vi "Multiplexer_sendsubvi.vi"(3 "error in (no error)":errorcluster, 4 "Position":i32 min=0 max=7, 5 "Enum":T1(ring), 6 "VISA resource name":refnum<visa-resource-name>) -> (0 "error out":errorcluster, 1 "Response":string="answ 0\rjmp 1\rla 200\rla 35010001\rla -562\rla 358\rla 1246\rla 2136\rla 3038\rla 3926\rla 4816\rla 5718\rla -562\rla 358\rla 1246\rla 2136\rla 3038\rla 3926\rla 4816\rla 5718\ra 1\rv -70\rdelay 600\rgohix \rdelay 50\rla -562\rm \rdelay 50\rend:53\r\n", 2 "VISA resource name out":refnum<visa-resource-name>)   [LabVIEW 2018]
panel:
  out "concatenated string":string="GPROGSEQ\r"
  out "bytes read":u32=222
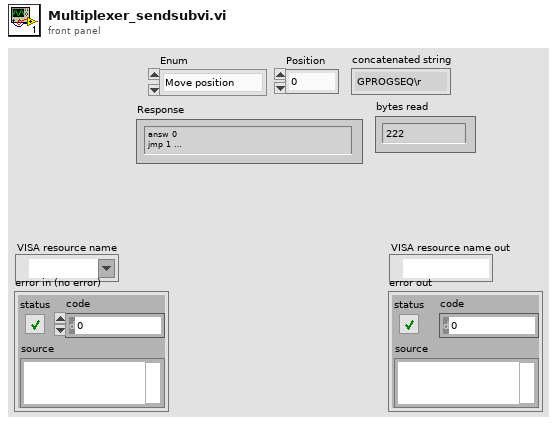
[diagram p1: front panel]
types:
  T1 = enum16{"Move position", "Get Status", "Get Program"}
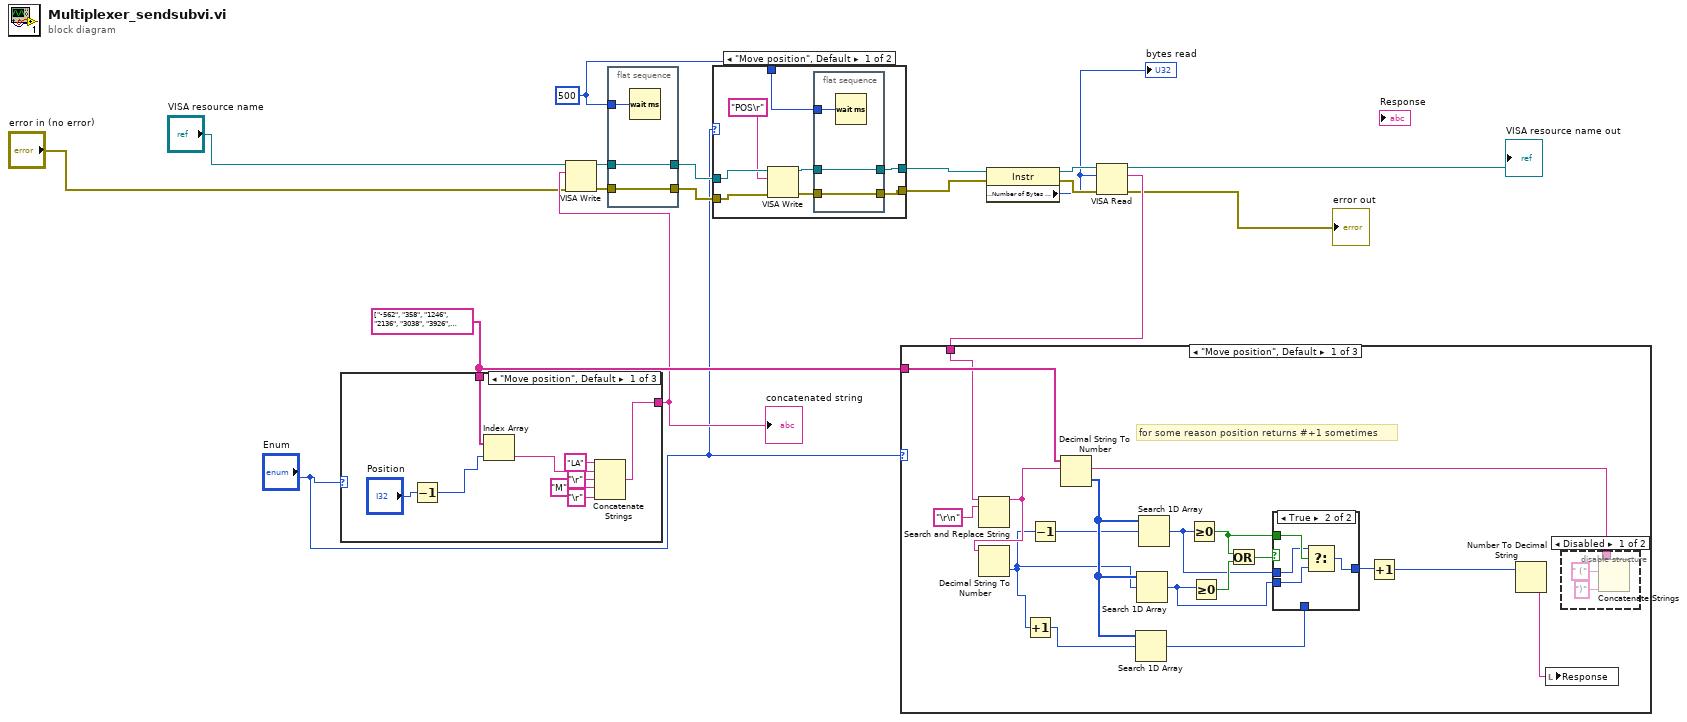
[diagram p0: block diagram]
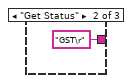
[diagram p7: hidden frame]
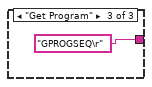
[diagram p8: hidden frame]
diagram:
  w12 = string[] ["-562", "358", "1246", "2136", "3038", "3926", "4816", "5718"]
  w7 = u32 500 ("delay before read (ms)")
  n1 = case shown="\"Move position\", Default" "Enum" {
    tunnel: [w22 "GST\r" "GPROGSEQ\r"] -> w11
    tunnel: w12 -> [w21 _ _]
    frame "Move position", Default {
      n2 = Decrement(x="Position") -> (x-1=w19:i32)
      n3 = Index Array(array=w21, index=w19) -> (element=w25:string)
      n4 = Concatenate Strings("LA" ("string"), w25, "\r" ("string"), "M" ("string"), "\r" ("string")) -> (w22:string)
    }
    frame "Get Status" {
    }
    frame "Get Program" {
    }
  }
  "concatenated string" <- w11
  n5 = VISA Write(VISA resource name="VISA resource name", write buffer=w11, error in (no error)="error in (no error)") -> (VISA resource name out=w17:refnum<visa-resource-name>, error out=w18:errorcluster)  [unwired: 1 out]
  n6 = flat-sequence {
    tunnel: w18 -> [w31]
    tunnel: [w31] -> w9
    tunnel: w17 -> [w30]
    tunnel: [w30] -> w10
    tunnel: w7 -> [w32]
    frame #0 {
      n7 = Wait (ms)(milliseconds to wait=w32) -> ()  [unwired: 1 out]
    }
  }
  n8 = case shown="\"Move position\", Default" "Enum" {
    tunnel: w10 -> [w40 w45]
    tunnel: w9 -> [w39 w44]
    tunnel: [w33 w44] -> w5
    tunnel: [w34 w45] -> w6
    tunnel: w7 -> [w37 _]
    frame "Move position", Default {
      n9 = VISA Write(VISA resource name=w40, write buffer="POS\r", error in (no error)=w39) -> (VISA resource name out=w36:refnum<visa-resource-name>, error out=w35:errorcluster)  [unwired: 1 out]
      n10 = flat-sequence {
        tunnel: w35 -> [w42]
        tunnel: [w42] -> w33
        tunnel: w36 -> [w41]
        tunnel: [w41] -> w34
        tunnel: w37 -> [w43]
        frame #0 {
          n11 = Wait (ms)(milliseconds to wait=w43) -> ()  [unwired: 1 out]
        }
      }
    }
    frame "Get Status" {
    }
  }
  n12 = property class="Instr"(reference=w6, error in=w5) -> (reference out=w16:refnum<visa-resource-name>, error out=w15:errorcluster, "Serial Settings:Number of Bytes at Serial Port"=w14:u32)
  "bytes read" <- w14
  n13 = VISA Read(VISA resource name=w16, byte count=w14, error in (no error)=w15) -> (VISA resource name out=→"VISA resource name out":refnum<visa-resource-name>, read buffer=w13:string, error out=→"error out":errorcluster)  [unwired: 1 out]
  n14 = case shown="\"Move position\", Default" "Enum" {
    tunnel: w13 -> [w49 _ _]
    tunnel: w12 -> [w50 _ _]
    frame "Move position", Default {
      # "for some reason position returns #+1 sometimes"
      n15 = Search and Replace String(input string=w49, search string="\r\n") -> (result string=w62:string)  [unwired: 6 in, 3 out]
      n16 = Decimal String To Number(string=w62) -> (number=w58:i32)  [unwired: 2 in, 1 out]
      n17 = Increment(x=w58) -> (x+1=w57:i32)
      n18 = Decrement(x=w58) -> (x-1=w59:i32)
      n19 = Decimal String To Number(string=w50) -> (number=w60:i32[])  [unwired: 2 in, 1 out]
      n20 = Search 1D Array(1D array=w60, element=w57) -> (index of element=w51:i32)  [unwired: 1 in]
      n21 = Search 1D Array(1D array=w60, element=w58) -> (index of element=w52:i32)  [unwired: 1 in]
      n22 = Search 1D Array(1D array=w60, element=w59) -> (index of element=w53:i32)  [unwired: 1 in]
      n23 = Greater Or Equal To 0?(x=w53) -> (x >= 0?=w54:bool)
      n24 = Greater Or Equal To 0?(x=w52) -> (x >= 0?=w56:bool)
      n25 = Or(x=w54, y=w56) -> (x .or. y?=w55:bool)
      n26 = case shown="True" w55 {
        tunnel: w54 -> [_ w70]
        tunnel: w53 -> [_ w69]
        tunnel: w52 -> [_ w68]
        tunnel: w51 -> [w66 _]
        tunnel: [w66 w67] -> w47
        frame False {
        }
        frame True {
          n27 = Select(t=w69, s=w70, f=w68) -> (s? t:f=w67:i32)
        }
      }
      n28 = Increment(x=w47) -> (x+1=w46:i32)
      n29 = Number To Decimal String(number=w46) -> (decimal integer string=w48:string)  [unwired: 1 in]
      n30 = local write "Response"(w48) -> ()
      n31 = disable-structure shown="Disabled" {
        disable-tunnel: w62 -> [w65 _]
        frame Disabled {
          n32 = Concatenate Strings(" (" ("string"), w65, ")" ("string")) -> ()  [unwired: 1 in, 1 out]
        }
        frame Enabled {
        }
      }
    }
    frame "Get Status" {
    }
    frame "Get Program" {
    }
  }
